vi "Begin.vi"(11 "Image Size":T1=enum."160x120") -> (0 "error out":errorcluster)   [LabVIEW 2011]
doc: "Called before other user functions, this VI is expected to open initial I/O refnums, load in file data, and do all program initialization. Notice that the <B>error out</B> terminal is simply used for data flow. Wiring it to other structures or subVIs ensures that this VI runs first."
uses:
  <vilib>/Rock Robotics/WPI/Camera/WPI_CameraImageSize.ctl
  <vilib>/Rock Robotics/SystemInterfaces/DIO/FPGA_DIOPWMChannel.ctl
  <vilib>/Rock Robotics/WPI/Joystick/WPI_JoystickDeviceEnum.ctl
  <vilib>/Rock Robotics/WPI/Camera/WPI_CameraWhite Balance Values.ctl
  <vilib>/Rock Robotics/WPI/Camera/WPI_CameraExposure Values.ctl
  <vilib>/Rock Robotics/WPI/Camera/WPI_CameraFrameRate.ctl
  <vilib>/Rock Robotics/SystemInterfaces/DIO/FPGA_DIORelayChannel.ctl
  <vilib>/Rock Robotics/WPI/RobotDrive/WPI_RobotDriveOpen2MotorWithJaguar.vi
panel:
  in  "Image Size 2":T1=enum."160x120"
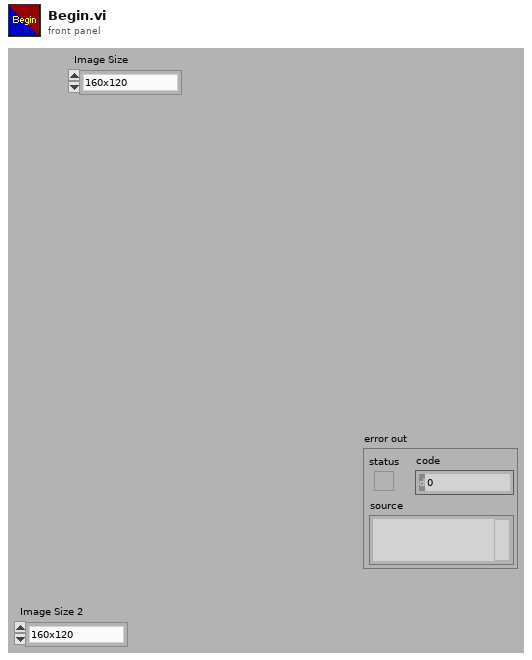
[diagram p1: front panel]
types:
  T1 = typedef "WPI_CameraImageSize.ctl" = enum16{"640x480", "320x240", "160x120"}
  T2 = typedef "FPGA_DIORelayChannel.ctl" = enum8{"Relay 1", "Relay 2", "Relay 3", "Relay 4", "Relay 5", "Relay 6", "Relay 7", "Relay 8", "Invalid"}
  T3 = typedef "WPI_CameraFrameRate.ctl" = u32
  T4 = typedef "WPI_CameraExposure Values.ctl" = enum16{"Auto", "Flicker-free 50 Hz", "Flicker-free 60 Hz", "Hold current"}
  T5 = typedef "WPI_CameraWhite Balance Values.ctl" = enum16{"Auto", "Fixed indoor", "Fixed outdoor 1", "Fixed outdoor 2", "Fixed fluorescent 1", "Fixed fluorescent 2", "Hold current"}
  T6 = typedef "WPI_JoystickDeviceEnum.ctl" = enum16{"USB 1", "USB 2", "USB 3", "USB 4", "Kinect 1", "Kinect 2"}
  T7 = typedef "FPGA_DIOPWMChannel.ctl" = enum8{"PWM 1", "PWM 2", "PWM 3", "PWM 4", "PWM 5", "PWM 6", "PWM 7", "PWM 8", "PWM 9", "PWM 10", "Invalid"}
  T8 = typedef "WPI_RelayDevRef.ctl" = cluster{"DevStatus":errorcluster, "Relay Channel":T2, "Digital Module":T9, "Relay Direction":T10}
  T9 = typedef "FPGA_TypedefDigitalModule.ctl" = enum16{"Digital Module 1", "Digital Module 2"}
  T10 = typedef "WPI_RelayDirection.ctl" = enum16{"Both directions", "Forward only", "Reverse only"}
  T11 = typedef "WPI_CameraDevRef.ctl" = cluster{"Camera Address":string, "CameraStatus":errorcluster, "Acquire Image Notifier":refnum<notifier>}
  T12 = typedef "WPI_RobotDriveDevRef.ctl" = cluster{"DevStatus":errorcluster, "Motors[]":T13[], "Square Inputs":bool, "Max Output":dbl, "Isochronous":bool}
  T13 = typedef "WPI_MotorControlDeviceRef.ctl" = cluster{"DeviceStatus":errorcluster, "Type":enum16{"PWM", "CAN"}, "PWM":cluster{"Digital Module":T9, "PWM Channel":T7, "DeadBand":T14}, "CAN":cluster{"Device Number":u8, "Control Mode":T15, "Semaphore":T16, "Max Vout":dbl}, "Invert":bool, "TransformRef":T17, "InvTransformRef":T17}
  T14 = typedef "WPI_PWMDeadband.ctl" = cluster{"Name":string, "maxPositivePwm":i32, "minPositivePwm":i32, "centerPwm":i32, "maxNegativePwm":i32, "minNegativePwm":i32, "angularRange":u16}
  T15 = typedef "WPI_CANJaguar_ControlMode.ctl" = enum8{"Percent VBus", "Current", "Speed", "Position", "Voltage"}
  T16 = typedef "Semaphore RefNum" = refnum<k1>
  T17 = typedef "WPI_PWMTransform_ConPane.ctl" = refnum<vi>
  T18 = typedef "WPI_JoystickDevRef.ctl" = cluster{"Device":T6}
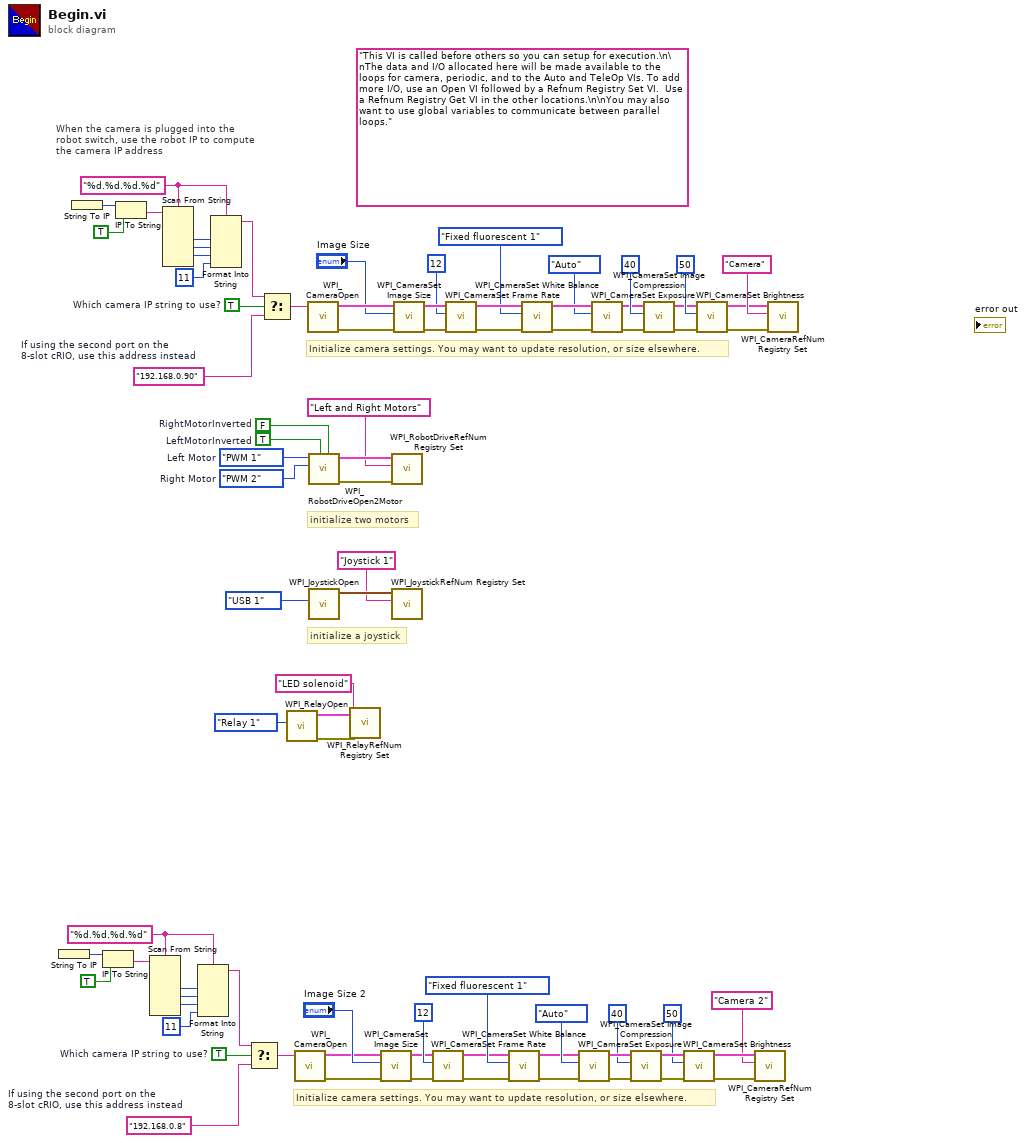
[diagram p0: block diagram]
diagram:
  w37 = TRUE  # Which camera IP string to use?
  w33 = "%d.%d.%d.%d" ("format string")
  w36 = "192.168.0.8"  # If using the second port on the 8-slot cRIO, use this address instead
  w38 = TRUE  # Which camera IP string to use?
  w42 = "%d.%d.%d.%d" ("format string")
  (unwired) "This VI is called before others so you can setup for execution.\n\nThe data and I/O allocated here will be made available to the loops for camera, periodic, and to the Auto and TeleOp VIs. To add more I/O, use an Open VI followed by a Refnum Registry Set VI.  Use a Refnum Registry Get VI in the other locations.\n\nYou may also want to use global variables to communicate between parallel loops."
  w54 = FPGA_DIOPWMChannel."PWM 2"  # Right Motor
  w55 = FPGA_DIOPWMChannel."PWM 1"  # Left Motor
  w39 = "192.168.0.90"  # If using the second port on the 8-slot cRIO, use this address instead
  w79 = TRUE  # LeftMotorInverted
  w80 = FALSE  # RightMotorInverted
  # "Initialize camera settings. You may want to update resolution, or size elsewhere."
  # "When the camera is plugged into the\nrobot switch, use the robot IP to compute\nthe camera IP address"
  # "initialize a joystick"
  # "initialize two motors"
  # "Initialize camera settings. You may want to update resolution, or size elsewhere."
  n1 = String To IP() -> (0:w26:u32)  [unwired: 1 in]
  n2 = String To IP() -> (0:w49:u32)  [unwired: 1 in]
  n3 = IP To String(1:TRUE ("dot notation? (F)"), 2:w26) -> (0:w28:string)
  n4 = IP To String(1:TRUE ("dot notation? (F)"), 2:w49) -> (0:w47:string)
  n5 = Scan From String(format string=w33, input string=w28) -> (output 1=w29:i32, output 2=w30:i32, output 3=w31:i32)  [unwired: 7 in, 3 out]
  n6 = Scan From String(format string=w42, input string=w47) -> (output 1=w46:i32, output 2=w45:i32, output 3=w44:i32)  [unwired: 7 in, 3 out]
  n7 = Format Into String(format string=w33, w29, w30, w31, 11 ("Compression")) -> (resulting string=w35:string)  [unwired: 2 in, 1 out]
  n8 = Format Into String(format string=w42, w46, w45, w44, 11 ("Compression")) -> (resulting string=w40:string)  [unwired: 2 in, 1 out]
  n9 = Select(t=w35, s=w37, f=w36) -> (s? t:f=w34:string)
  n10 = Select(t=w40, s=w38, f=w39) -> (s? t:f=w41:string)
  n11 = call <vilib>:"WPI_RelayOpen.vi"("Relay Channel"=FPGA_DIORelayChannel."Relay 1") -> ("error out"=w4:errorcluster, "RelayDevRef"=w3:T8)  [unwired: 9 in]
  n12 = call <vilib>:"WPI_CameraOpen.vi"("Camera Address"=w34) -> ("error out"=w14:errorcluster, "CameraDevRef"=w13:T11)  [unwired: 1 in, 8 out]
  n13 = call <vilib>:"WPI_CameraOpen.vi"("Camera Address"=w41) -> ("error out"=w64:errorcluster, "CameraDevRef"=w65:T11)  [unwired: 1 in, 8 out]
  n14 = call-poly <vilib>:"WPI_RobotDriveOpen2Motor.vi"("Right Motor Inverted"=w80, "Left Motor Inverted"=w79, "Right Motor"=w54, "Left Motor"=w55) -> ("error out"=w73:errorcluster, "RobotDriveDevRef"=w77:T12)  [unwired: 1 in, 5 out]
  n15 = call <vilib>:"WPI_JoystickOpen.vi"("JoystickDevice"=WPI_JoystickDeviceEnum."USB 1") -> ("JoystickDevRef"=w75:T18)  [unwired: 10 out]
  n16 = call <vilib>:"WPI_RelayRefNum Registry Set.vi"("error in (no error)"=w4, "refnum name"="LED solenoid", "RelayDevRef"=w3) -> ()  [unwired: 7 in, 2 out]
  n17 = call <vilib>:"WPI_CameraSet Image Size.vi"("error in (no error)"=w14, "Image Size"="Image Size 2", "CameraDevRef"=w13) -> ("error out"=w15:errorcluster, "CameraDevRef Out"=w12:T11)  [unwired: 7 out]
  n18 = call <vilib>:"WPI_RobotDriveRefNum Registry Set.vi"("error in (no error)"=w73, "refnum name"="Left and Right Motors", "RobotDriveDevRef"=w77) -> ()  [unwired: 9 out]
  n19 = call <vilib>:"WPI_JoystickRefNum Registry Set.vi"("refnum name"="Joystick 1", "JoystickDevRef"=w75) -> ()  [unwired: 1 in, 9 out]
  n20 = call <vilib>:"WPI_CameraSet Image Size.vi"("error in (no error)"=w64, "Image Size"="Image Size", "CameraDevRef"=w65) -> ("error out"=w63:errorcluster, "CameraDevRef Out"=w66:T11)  [unwired: 7 out]
  n21 = call <vilib>:"WPI_CameraSet Frame Rate.vi"("error in (no error)"=w15, "Frame Rate (fps)"=T3 12, "CameraDevRef"=w12) -> ("error out"=w16:errorcluster, "CameraDevRef Out"=w10:T11)  [unwired: 7 out]
  n22 = call <vilib>:"WPI_CameraSet Frame Rate.vi"("error in (no error)"=w63, "Frame Rate (fps)"=T3 12, "CameraDevRef"=w66) -> ("error out"=w62:errorcluster, "CameraDevRef Out"=w68:T11)  [unwired: 7 out]
  n23 = call <vilib>:"WPI_CameraSet White Balance.vi"("error in (no error)"=w16, "White Balance"=WPI_CameraWhite_Balance_Values."Fixed fluorescent 1", "CameraDevRef"=w10) -> ("error out"=w17:errorcluster, "CameraDevRef Out"=w11:T11)  [unwired: 7 out]
  n24 = call <vilib>:"WPI_CameraSet White Balance.vi"("error in (no error)"=w62, "White Balance"=WPI_CameraWhite_Balance_Values."Fixed fluorescent 1", "CameraDevRef"=w68) -> ("error out"=w61:errorcluster, "CameraDevRef Out"=w67:T11)  [unwired: 7 out]
  n25 = call <vilib>:"WPI_CameraSet Exposure.vi"("error in (no error)"=w17, "Exposure"=WPI_CameraExposure_Values."Auto", "CameraDevRef"=w11) -> ("error out"=w18:errorcluster, "CameraDevRef Out"=w8:T11)  [unwired: 7 out]
  n26 = call <vilib>:"WPI_CameraSet Exposure.vi"("error in (no error)"=w61, "Exposure"=WPI_CameraExposure_Values."Auto", "CameraDevRef"=w67) -> ("error out"=w60:errorcluster, "CameraDevRef Out"=w70:T11)  [unwired: 7 out]
  n27 = call <vilib>:"WPI_CameraSet Image Compression.vi"("error in (no error)"=w18, "Compression"=40, "CameraDevRef"=w8) -> ("error out"=w19:errorcluster, "CameraDevRef Out"=w9:T11)  [unwired: 7 out]
  n28 = call <vilib>:"WPI_CameraSet Image Compression.vi"("error in (no error)"=w60, "Compression"=40, "CameraDevRef"=w70) -> ("error out"=w59:errorcluster, "CameraDevRef Out"=w69:T11)  [unwired: 7 out]
  n29 = call <vilib>:"WPI_CameraSet Brightness.vi"("error in (no error)"=w19, "Brightness"=50, "CameraDevRef"=w9) -> ("error out"=w21:errorcluster, "CameraDevRef Out"=w20:T11)  [unwired: 7 out]
  n30 = call <vilib>:"WPI_CameraSet Brightness.vi"("error in (no error)"=w59, "Brightness"=50, "CameraDevRef"=w69) -> ("error out"=w57:errorcluster, "CameraDevRef Out"=w58:T11)  [unwired: 7 out]
  n31 = call <vilib>:"WPI_CameraRefNum Registry Set.vi"("error in (no error)"=w21, "refnum name"="Camera 2", "CameraDevRef"=w20) -> ()  [unwired: 9 out]
  n32 = call <vilib>:"WPI_CameraRefNum Registry Set.vi"("error in (no error)"=w57, "refnum name"="Camera", "CameraDevRef"=w58) -> ()  [unwired: 9 out]
